vi "Bundle Script_Named (Un)Bundler Insert.vi"(4 "Hide Full Names":bool=TRUE, 6 "Dialog Choice":enum32{"Choice 1", "Choice 2"}(radio), 8 "error in":errorcluster, 10 "Selected Items (tags)":string[](array[string]), 11 "Affected Items":T1) -> (0 "error out":errorcluster, 2 "Objects":refnum<vi>[](array[refnum]))   [LabVIEW 2023]
uses:
  top/BundleMagic.ctl
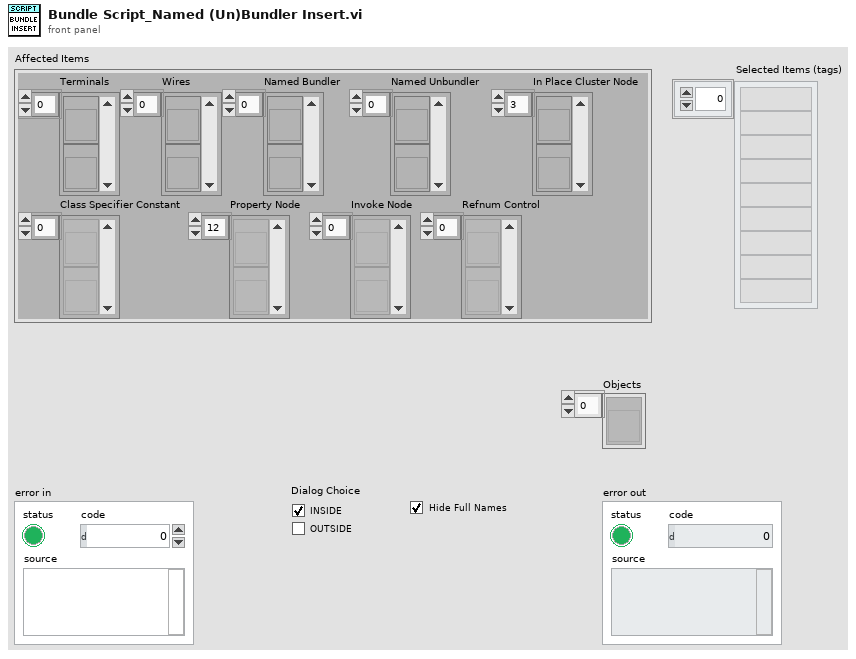
[diagram p1: front panel]
types:
  T1 = typedef "BundleMagic.ctl" = cluster{"Terminals":refnum<vi>[], "Wires":refnum<vi>[], "Named Bundler":refnum<vi>[], "Named Unbundler":refnum<vi>[], "In Place Cluster Node":refnum<vi>[], "Class Specifier Constant":refnum<vi>[], "Property Node":refnum<vi>[], "Invoke Node":refnum<vi>[], "Refnum Control":refnum<vi>[]}
  T2 = enum16{"Named Bundler", "Named Unbundler", "In Place", "None"}
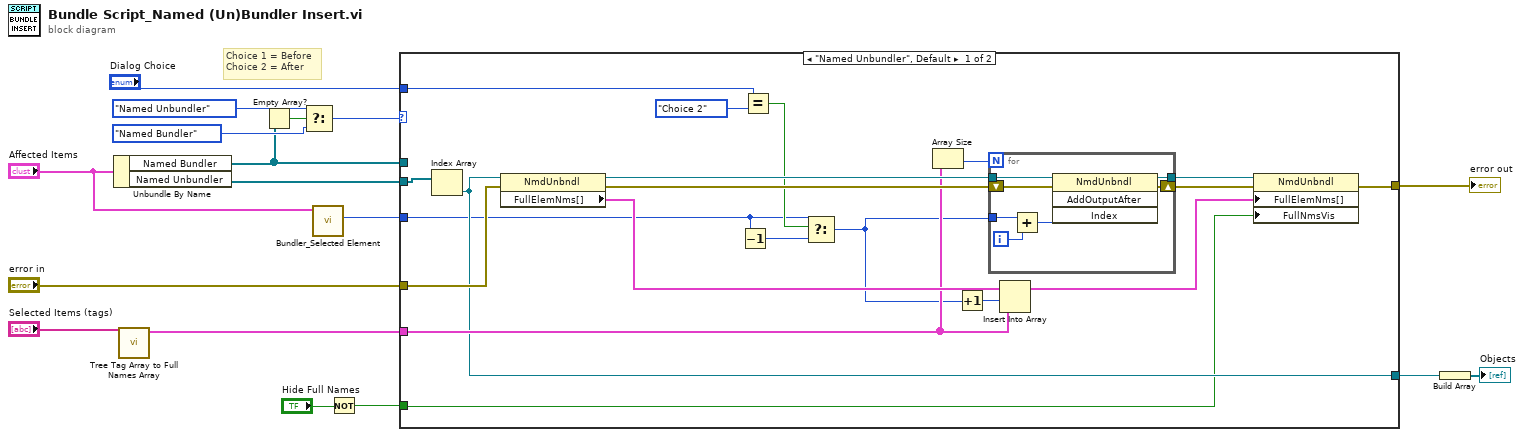
[diagram p0: block diagram]
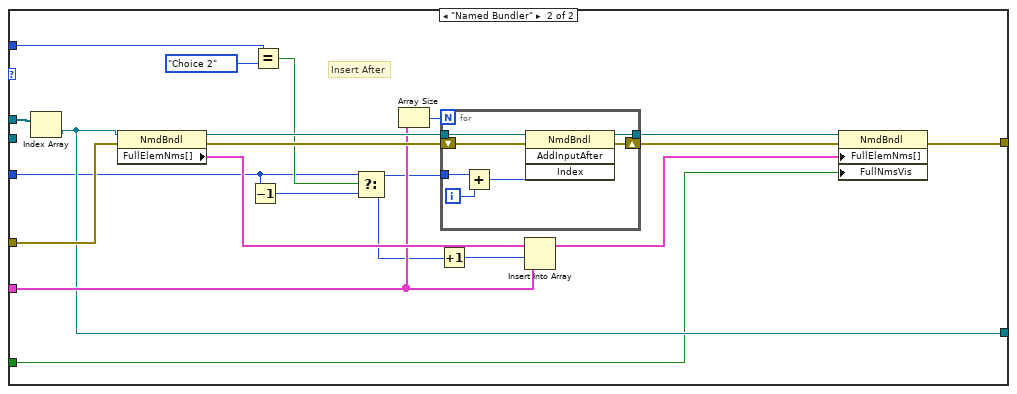
[diagram p2: hidden frame]
diagram:
  # "Choice 1 = Before\nChoice 2 = After"
  n1 = Unbundle By Name("Affected Items") -> ("Named Bundler"=w11:refnum<vi>[], "Named Unbundler"=w12:refnum<vi>[])
  n2 = call "Tree Tag Array to Full Names Array.vi"("Selected Items Tags"="Selected Items (tags)") -> ("Tree Item Values (nested form)"=w5:cluster{"Array":string[]}[])  [unwired: 6 in, 4 out]
  n3 = Empty Array?(array=w11) -> (empty?=w16:bool)
  n4 = Select(t=T2."Named Unbundler" ("Bundler Type"), s=w16, f=T2."Named Bundler" ("Bundler Type")) -> (s? t:f=w13:T2)
  n5 = call "Bundler_Selected Element.vi"("Affected Items"="Affected Items") -> ("index of element"=w3:i32)  [unwired: 4 in, 6 out]
  n6 = Not(x="Hide Full Names") -> (.not. x?=w1:bool)
  n7 = case shown="\"Named Unbundler\", Default" w13 {
    tunnel: "error in" -> [w37 w64]
    tunnel: [w29 w56] -> w9
    tunnel: w5 -> [w31 w58]
    tunnel: "Dialog Choice" -> [w21 w48]
    tunnel: w12 -> [w28 _]
    tunnel: w11 -> [_ w55]
    tunnel: [w27 w54] -> w10
    tunnel: w3 -> [w19 w46]
    tunnel: w1 -> [w18 w45]
    frame "Named Unbundler", Default {
      n8 = Index Array(array=w28) -> (element=w27:refnum<vi>)  [unwired: 1 in]
      n9 = property class="NmdUnbndl"(reference=w27, error in=w37) -> (reference out=w33:refnum<vi>, error out=w35:errorcluster, "FullElemNms[]"=w32:cluster{string[]}[])
      n10 = Decrement(x=w19) -> (x-1=w22:i32)
      n11 = Equal?(x=w21, y=enum32{"Choice 1", "Choice 2"}."Choice 2" ("Dialog Choice")) -> (x = y?=w23:bool)
      n12 = Select(t=w19, s=w23, f=w22) -> (s? t:f=w20:i32)
      n13 = Array Size(array=w31) -> (size(s)=w26:i32)
      n14 = Increment(x=w20) -> (x+1=w25:i32)
      n15 = for {
        N: w26 -> [_]
        shift-right: [w42] -> w34
        shift-left: w35 -> [w43]
        tunnel: w33 -> [w41]
        tunnel: [w44] -> w36
        tunnel: w20 -> [w39]
        i -> [w38]
        n16 = Add(x=w39, y=w38) -> (x+y=w40:i32)
        n17 = invoke class="NmdUnbndl" method="AddOutputAfter"(reference=w41, error in=w43, "Index"=w40) -> (reference out=w44:refnum<vi>, error out=w42:errorcluster)  [unwired: 1 in, 2 out]
      }
      n18 = Insert Into Array(array=w32, index=w25, new element=w31) -> (w30:cluster{string[]}[])
      n19 = property class="NmdUnbndl"(reference=w36, error in=w34, "FullElemNms[]"=w30, "FullNmsVis"=w18) -> (error out=w29:errorcluster)  [unwired: 1 out]
    }
    frame "Named Bundler" {
      # "Insert After"
      n20 = Index Array(array=w55) -> (element=w54:refnum<vi>)  [unwired: 1 in]
      n21 = property class="NmdBndl"(reference=w54, error in=w64) -> (reference out=w60:refnum<vi>, error out=w62:errorcluster, "FullElemNms[]"=w59:cluster{string[]}[])
      n22 = Decrement(x=w46) -> (x-1=w50:i32)
      n23 = Equal?(x=w48, y=enum32{"Choice 1", "Choice 2"}."Choice 2" ("Dialog Choice")) -> (x = y?=w51:bool)
      n24 = Select(t=w46, s=w51, f=w50) -> (s? t:f=w47:i32)
      n25 = Array Size(array=w58) -> (size(s)=w53:i32)
      n26 = Increment(x=w47) -> (x+1=w52:i32)
      n27 = for {
        N: w53 -> [_]
        shift-right: [w69] -> w61
        shift-left: w62 -> [w70]
        tunnel: w60 -> [w68]
        tunnel: [w71] -> w63
        tunnel: w47 -> [w66]
        i -> [w65]
        n28 = Add(x=w66, y=w65) -> (x+y=w67:i32)
        n29 = invoke class="NmdBndl" method="AddInputAfter"(reference=w68, error in=w70, "Index"=w67) -> (reference out=w71:refnum<vi>, error out=w69:errorcluster)  [unwired: 1 in, 2 out]
      }
      n30 = Insert Into Array(array=w59, index=w52, new element=w58) -> (w57:cluster{string[]}[])
      n31 = property class="NmdBndl"(reference=w63, error in=w61, "FullElemNms[]"=w57, "FullNmsVis"=w45) -> (error out=w56:errorcluster)  [unwired: 1 out]
    }
  }
  "error out" <- w9
  n32 = Build Array(w10) -> (→"Objects":refnum<vi>[])
